vi "Data Acquisition subVI.vi"(8 "Numeric in":i32) -> (3 "Numeric out":dbl)   [LabVIEW 2014]
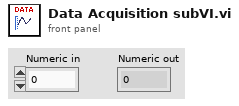
[diagram p1: front panel]
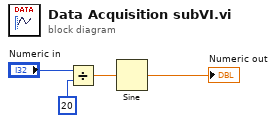
[diagram p0: block diagram]
diagram:
  n1 = Divide(x="Numeric in", y=20) -> (x/y=w2:dbl)
  n2 = Sine(x=w2) -> (sin(x)=→"Numeric out":dbl)
